vi "U Boat main 3.vi"() -> ()   [LabVIEW 2013]
uses:
  <vilib>/Utility/inputDevices.llb/closeJoystick.vi
  <vilib>/Utility/inputDevices.llb/joystickAcquire.vi
panel:
  out "Valid ?":bool
  out "Boat Nav Data":T1
  out "data rec'd":string="$,G,43,13,230,P,10,20,120,T,10,10,330,L,14,36,110,A,3,5,B,7,8,C,16,20,D,-1,-1,S,08,12,234\r"
  out "UDP Time Out?":bool
  out "J":u16
  out "R":u16
  out "M":u16
  out "Battery Volts":dbl
  out "Wind Direction":dbl
  out "Wind Speed":dbl
  out "Tilt":dbl
  out "Running?":bool
  in  "Jib Offset":i16 min=-100 max=100 step=1
  in  "Main Offset":i16 min=-100 max=100 step=1
  in  "Manual?":bool=TRUE
  out "Manual Out":i32[](array[numeric])
  in  "VISA resource name":refnum<visa-resource-name>="COM3"
  out "XBee ?":bool
  in  "String":string="$CR1500M1500J1500\n"
  out "bytes written":u32
  out "return count":u32
  out "String Received":string
  in  "Rudder\nOffset":i16 min=-100 max=100 step=1
  out "Jib Sheet":u16=1500
  out "Main sheet":u16=1500
  out "Rudder":u16=1500
  out "error out":errorcluster
  in  "stop":bool
  # "Raw data from\ncontroller"
  # "Values without offset"
  # "Servo Offsets"
  # "Values sent"
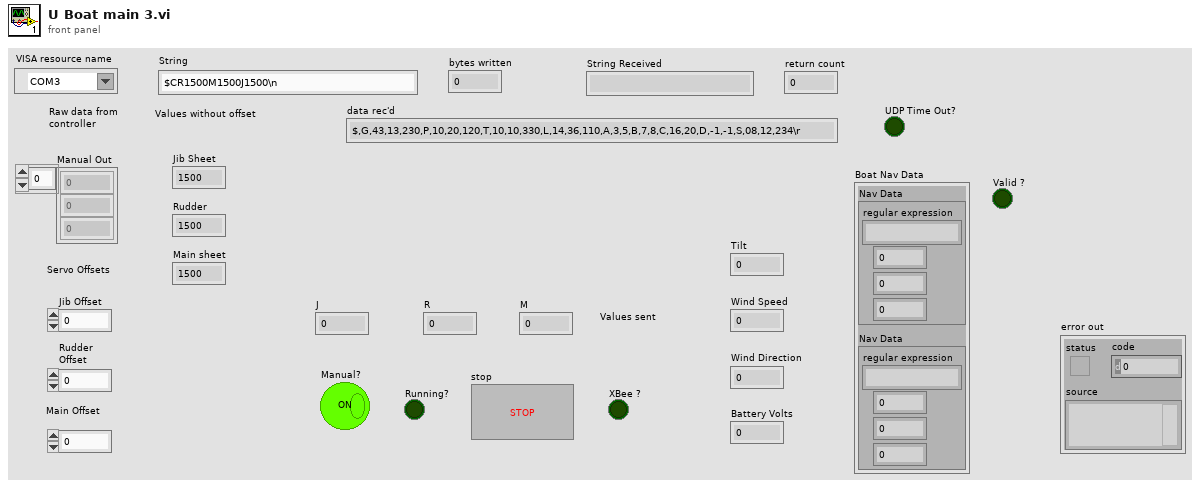
[diagram p1: front panel]
types:
  T1 = cluster{"Nav Data":cluster{"regular expression":string, i32, i32, i32}, "Nav Data":cluster{"regular expression":string, i32, i32, i32}}
  T2 = cluster{"X axis":i32, "Y axis":i32, "Z axis":i32, "X axis rotation":i32, "Y axis rotation":i32, "Z axis rotation":i32, "U axis":i32, "V axis":i32}
  T3 = cluster{"button 1":bool, "button 2":bool, "button 3":bool, "button 4":bool, "button 5":bool, "button 6":bool, "button 7":bool, "button 8":bool, "button 9":bool, "button 10":bool, "button 11":bool, "button 12":bool, "button 13":bool, "button 14":bool, "button 15":bool, "button 16":bool, "button 17":bool, "button 18":bool, "button 19":bool, "button 20":bool, "button 21":bool, "button 22":bool, "button 23":bool, "button 24":bool, "button 25":bool, "button 26":bool, "button 27":bool, "button 28":bool, "button 29":bool, "button 30":bool, "button 31":bool, "button 32":bool}
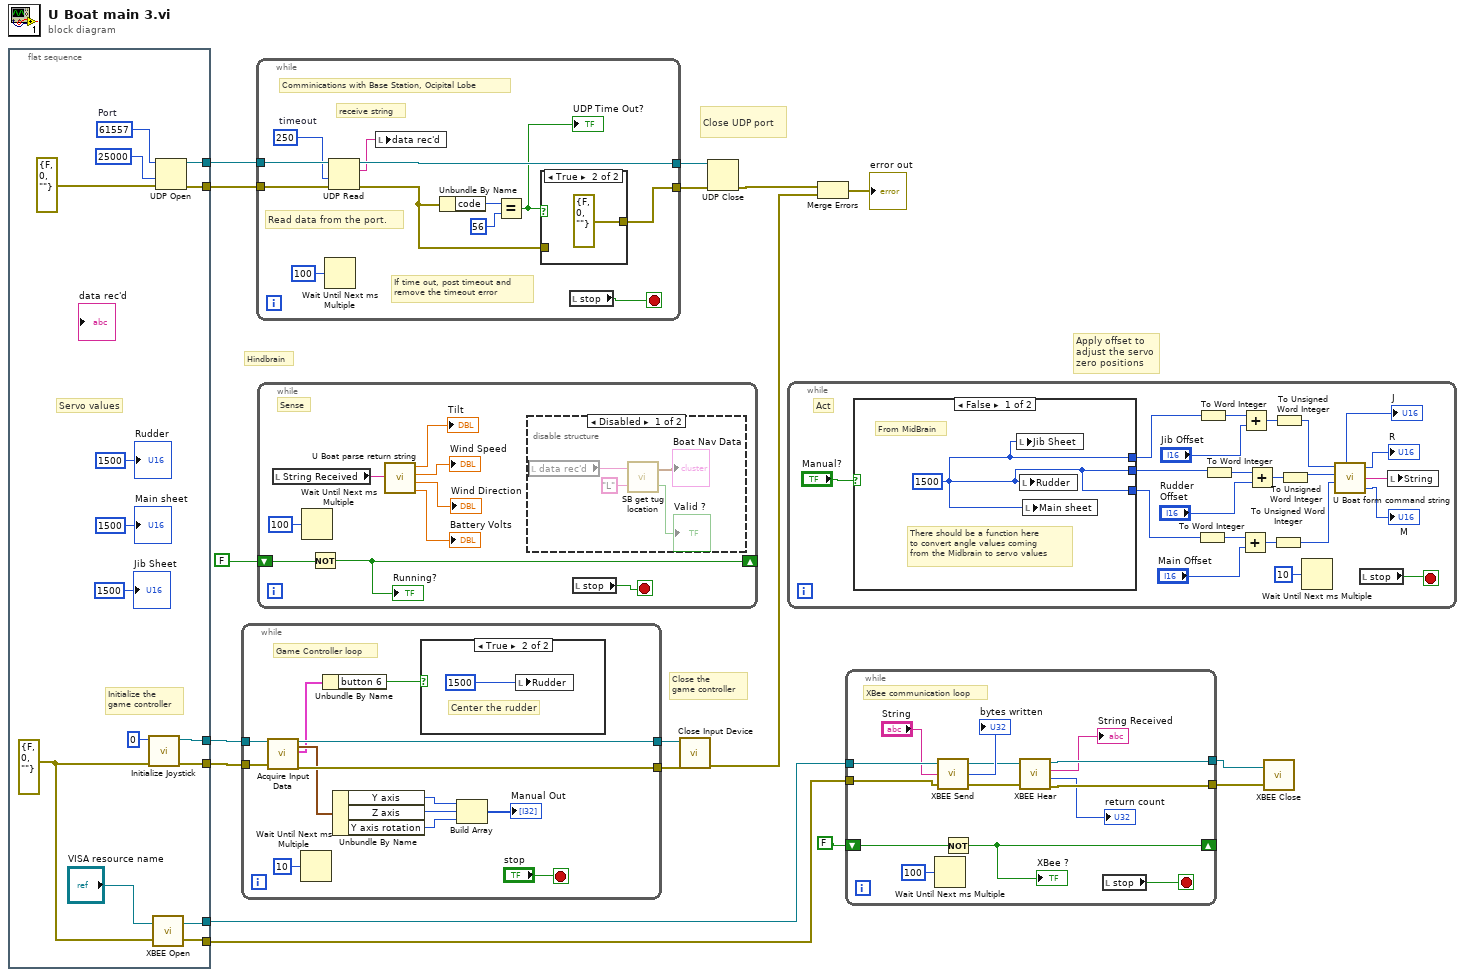
[diagram p0: block diagram]
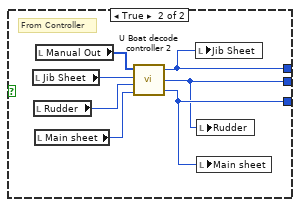
[diagram p3: hidden frame]
diagram:
  # "Close UDP port"
  # "Apply offset to \nadjust the servo \nzero positions"
  # "Hindbrain"
  # "Close the\ngame controller"
  n1 = flat-sequence {
    tunnel: [w31] -> w17
    tunnel: [w30] -> w15
    tunnel: [w28] -> w12
    tunnel: [w27] -> w11
    tunnel: [w20] -> w6
    tunnel: [w19] -> w5
    frame #0 {
      w21 = u16 61557  # Port
      w23 = errorcluster {"status"=FALSE, "code"=0, "source"=""} ("error in (no error)")
      # "Servo values"
      # "Initialize the\ngame controller"
      n2 = call <vilib>:"Initialize Joystick.vi"("error in (no error)"=w23, "device index"=0) -> ("error out"=w30:errorcluster, "device ID"=w31:refnum<k1>)  [unwired: 8 in]
      n3 = call "XBEE Open.vi"("error in"=w23, "VISA resource name"="VISA resource name") -> ("error out"=w27:errorcluster, "VISA resource name out"=w28:refnum<visa-resource-name>)
      n4 = UDP Open(8:errorcluster {"status"=FALSE, "code"=0, "source"=""} ("error in (no error)"), 9:25000 ("timeout ms (25000)"), 11:w21) -> (port=w20:refnum<k16>, 0:w19:errorcluster)  [unwired: 2 in, 1 out]
      "Rudder" <- u16 1500 ("MRudder")
      "Main sheet" <- u16 1500 ("MRudder")
      "Jib Sheet" <- u16 1500 ("MRudder")
    }
  }
  n5 = while {
    tunnel: w17 -> [w45]
    tunnel: [w44] -> w16
    tunnel: w15 -> [w43]
    tunnel: [w42] -> w4
    stop <- "stop" stop-if-true
    # "Game Controller loop"
    n6 = call-poly <vilib>:"Acquire Input Data.vi"("device ID"=w45, "error in (no error)"=w43) -> ("device ID"=w44:refnum<k1>, "axis info"=w39:T2, "button info"=w34:T3, "error out"=w42:errorcluster)  [unwired: 13 in, 1 out]
    n7 = Wait Until Next ms Multiple(millisecond multiple=u32 10) -> ()  [unwired: 1 out]
    n8 = Unbundle By Name(w34) -> ("button 6"=w33:bool)
    n9 = Unbundle By Name(w39) -> ("Y axis"=w38:i32, "Z axis"=w37:i32, "Y axis rotation"=w36:i32)
    n10 = case shown="True" w33 {
      frame False {
        # "Do nothing"
      }
      frame True {
        # "Center the rudder"
        n11 = local write "Rudder"(u16 1500) -> ()
      }
    }
    n12 = Build Array(w38, w37, w36) -> (→"Manual Out":i32[])
  }
  n13 = while {
    tunnel: w5 -> [w58]
    tunnel: w6 -> [w57]
    tunnel: [w56] -> w8
    tunnel: [w51] -> w7
    stop <- w47 stop-if-true
    w50 = 250  # timeout
    # "Comminications with Base Station, Ocipital Lobe"
    # "receive string"
    # "If time out, post timeout and\nremove the timeout error"
    # "Read data from the port."
    n14 = Wait Until Next ms Multiple(millisecond multiple=u32 100) -> ()  [unwired: 1 out]
    n15 = UDP Read(connection ID=w57, timeout ms (25000)=w50, 8:w58) -> (data out=w49:string, error out=w52:errorcluster, 3:w56:refnum<k16>)  [unwired: 1 in, 2 out]
    n16 = local write "data rec'd"(w49) -> ()
    n17 = Unbundle By Name(w52) -> ("code"=w55:i32)
    n18 = Equal?(x=w55, y=56) -> (x = y?=w53:bool)
    "UDP Time Out?" <- w53
    n19 = case shown="True" w53 {
      tunnel: [w59 errorcluster {"status"=FALSE, "code"=0, "source"=""} ("error out")] -> w51
      tunnel: w52 -> [w59 _]
      frame False {
      }
      frame True {
      }
    }
    n20 = local read "stop"() -> (w47:bool)
  }
  n21 = while {
    shift-right: [w66] -> _
    shift-left: FALSE -> [w67]
    stop <- w69 stop-if-true
    # "Sense"
    n22 = local read "String Received"() -> (w65:string)
    n23 = Wait Until Next ms Multiple(millisecond multiple=u32 100) -> ()  [unwired: 1 out]
    n24 = Not(x=w67) -> (.not. x?=w66:bool)
    "Running?" <- w66
    n25 = call "U Boat parse return string.vi"("Return String"=w65) -> ("Tilt"=→"Tilt":dbl, "Wind Speed"=→"Wind Speed":dbl, "Wind Direction"=→"Wind Direction":dbl, "Battery Volts"=→"Battery Volts":dbl)
    n26 = disable-structure shown="Disabled" {
      frame Disabled {
        n27 = local read "data rec'd"() -> (w70:string)
        n28 = call "SB get tug location.vi"("Tug"="L", "Nav String"=w70) -> ("Valid ?"=→"Valid ?":bool, "Tug Nav Data"=→"Boat Nav Data":cluster{"y":i32, "y":i32})
      }
      frame Enabled {
      }
    }
    n29 = local read "stop"() -> (w69:bool)
  }
  n30 = call-poly <vilib>:"Close Input Device.vi"("error in (no error)"=w4, "device ID"=w16) -> ("error out"=w2:errorcluster)  [unwired: 8 in]
  n31 = UDP Close(connection ID=w8, 8:w7) -> (error out=w1:errorcluster)  [unwired: 1 out]
  n32 = while {
    stop <- w95 stop-if-true
    # "Act"
    n33 = case shown="False" "Manual?" {
      tunnel: [w96 w100] -> w87
      tunnel: [w96 w98] -> w90
      tunnel: [w96 w99] -> w81
      frame False {
        w96 = u16 1500 ("Jib Sheet")
        # "There should be a function here\nto convert angle values coming\nfrom the Midbrain to servo values"
        # "From MidBrain"
        n34 = local write "Jib Sheet"(w96) -> ()
        n35 = local write "Rudder"(w96) -> ()
        n36 = local write "Main sheet"(w96) -> ()
      }
      frame True {
        # "From Controller"
        n37 = local read "Jib Sheet"() -> (w102:u16)
        n38 = local read "Rudder"() -> (w97:u16)
        n39 = local read "Main sheet"() -> (w103:u16)
        n40 = local read "Manual Out"() -> (w101:i32[])
        n41 = call "U Boat decode controller 2.vi"("Main sheet In"=w103, "Rudder In"=w97, "Jib Sheet In"=w102, "Manual In"=w101) -> ("Main sheet Out"=w99:u16, "Rudder Out"=w98:u16, "Jib Steet Out"=w100:u16)
        n42 = local write "Jib Sheet"(w100) -> ()
        n43 = local write "Rudder"(w98) -> ()
        n44 = local write "Main sheet"(w99) -> ()
      }
    }
    n45 = To Word Integer(number=w81) -> (16bit integer=w82:i16)
    n46 = To Word Integer(number=w87) -> (16bit integer=w88:i16)
    n47 = To Word Integer(number=w90) -> (16bit integer=w92:i16)
    n48 = Add(x=w82, y="Main Offset") -> (x+y=w83:i16)
    n49 = Add(x=w88, y="Jib Offset") -> (x+y=w89:i16)
    n50 = Add(x=w92, y="Rudder\nOffset") -> (x+y=w91:i16)
    n51 = To Unsigned Word Integer(number=w83) -> (unsigned 16bit integer=w78:u16)
    n52 = To Unsigned Word Integer(number=w89) -> (unsigned 16bit integer=w80:u16)
    n53 = To Unsigned Word Integer(number=w91) -> (unsigned 16bit integer=w79:u16)
    n54 = Wait Until Next ms Multiple(millisecond multiple=u32 10) -> ()  [unwired: 1 out]
    n55 = call "U Boat form command string.vi"("Jib Sheet"=w80, "Rudder"=w79, "Main sheet"=w78) -> ("Jib"=→"J":u16, "Rudder"=→"R":u16, "String"=w77:string, "Main"=→"M":u16)  [unwired: 1 in]
    n56 = local read "stop"() -> (w95:bool)
    n57 = local write "String"(w77) -> ()
  }
  n58 = Merge Errors(w1, w2) -> (→"error out":errorcluster)
  n59 = while {
    tunnel: w12 -> [w117]
    tunnel: w11 -> [w116]
    tunnel: [w111] -> w14
    tunnel: [w110] -> w13
    shift-right: [w114] -> _
    shift-left: FALSE -> [w115]
    stop <- w104 stop-if-true
    # "XBee communication loop"
    n60 = Wait Until Next ms Multiple(millisecond multiple=u32 100) -> ()  [unwired: 1 out]
    n61 = call "XBEE Send.vi"("error in (no error)"=w116, "String"="String", "VISA resource name"=w117) -> ("error out"=w107:errorcluster, "return count"=→"bytes written":u32, "VISA resource name out"=w108:refnum<visa-resource-name>)
    n62 = Not(x=w115) -> (.not. x?=w114:bool)
    "XBee ?" <- w114
    n63 = call "XBEE Hear.vi"("VISA resource name"=w108, "error in (no error)"=w107) -> ("VISA resource name out"=w111:refnum<visa-resource-name>, "String Received"=→"String Received":string, "return count"=→"return count":u32, "error out"=w110:errorcluster)
    n64 = local read "stop"() -> (w104:bool)
  }
  n65 = call "XBEE Close.vi"("error in (no error)"=w13, "VISA resource name"=w14) -> ()
